vi "FreqSel.vi"(5 "FreqSelRing":u16(ring)=1 items=["0.8 ms", "1.0 ms", "1.6 ms", "3.2 ms", "6.4 ms"]) -> (0 "set sample time [s]":sgl, 1 "actual T_DAQ [ms]":dbl, 2 "f_DAQ [kHz]":dbl, 3 "ModeHex":u16, 4 "FreqHex":u16)   [LabVIEW 2014]
panel:
  out "Hex2Decimal":dbl
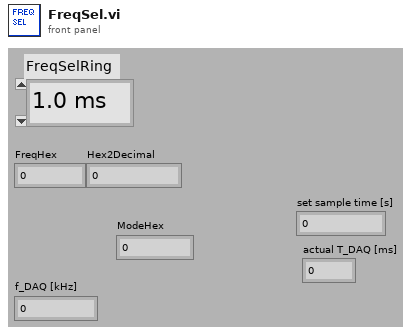
[diagram p1: front panel]
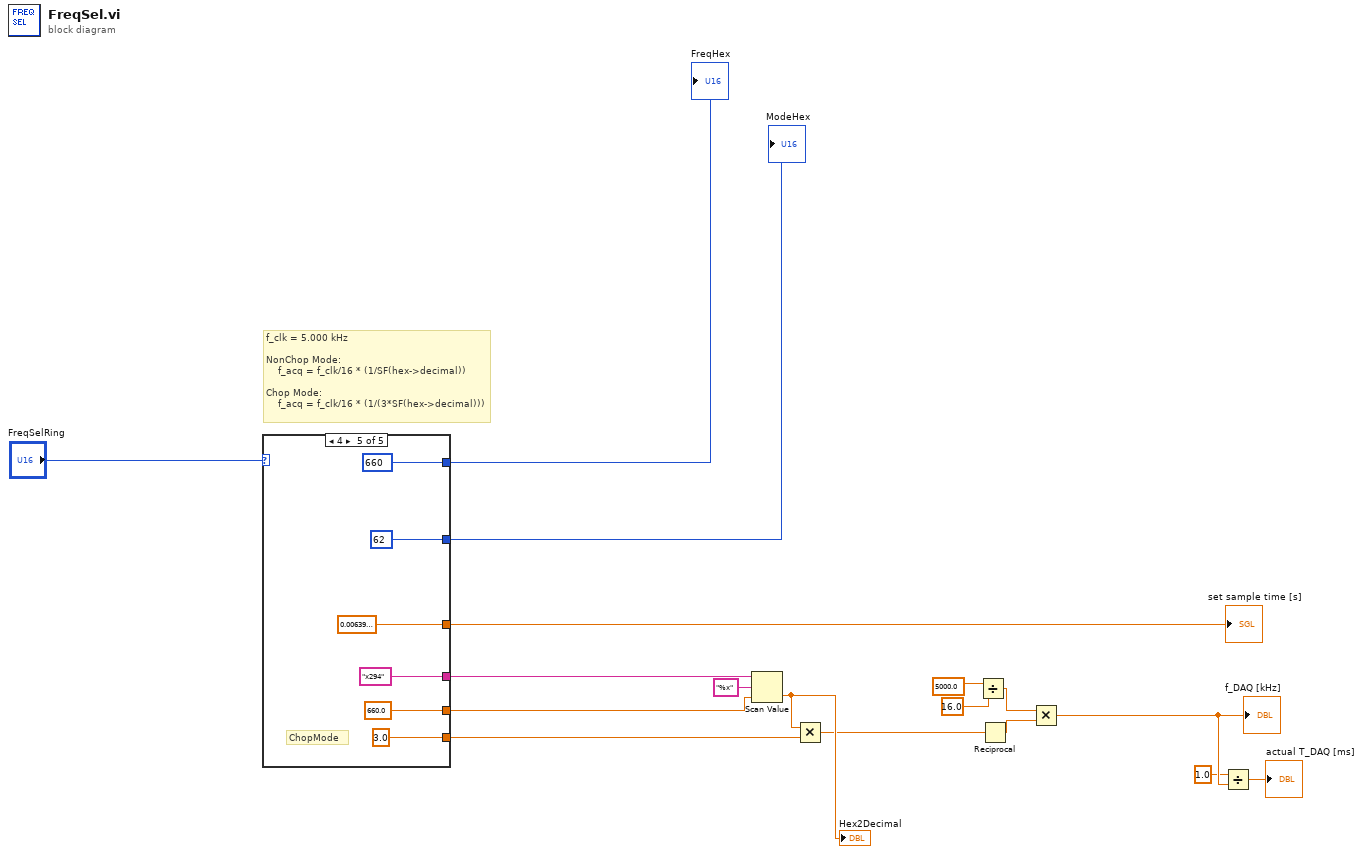
[diagram p0: block diagram]
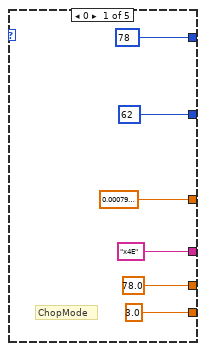
[diagram p2: hidden frame]
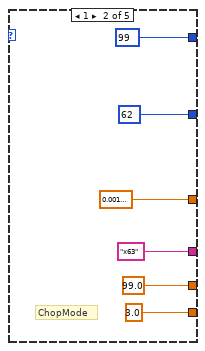
[diagram p3: hidden frame]
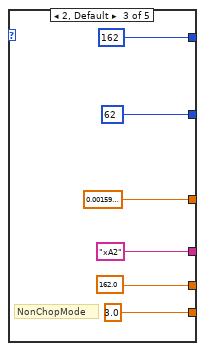
[diagram p4: hidden frame]
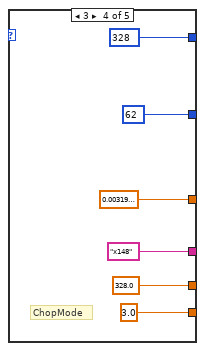
[diagram p5: hidden frame]
diagram:
  # "f_clk = 5.000 kHz\n\nNonChop Mode:\n    f_acq = f_clk/16 * (1/SF(hex->decimal))\n\nChop Mode:\n    f_acq = f_clk/16 * (1/(3*SF(hex->decimal)))"
  n1 = case shown="4" "FreqSelRing" {
    tunnel: [u16 78 ("frequenz") u16 99 ("frequenz") u8 162 ("frequenz") u16 328 ("frequenz") u16 660 ("frequenz")] -> w17
    tunnel: [u16 62 ("t") u16 62 ("t") u16 62 ("t") u16 62 ("t") u16 62 ("t")] -> w16
    tunnel: [sgl 0.0008 sgl 0.001 sgl 0.0016 sgl 0.0032 sgl 0.0064] -> w14
    tunnel: ["x4E" ("string") "x63" ("string") "xA2" ("string") "x148" ("string") "x294" ("string")] -> w3
    tunnel: [78.0 ("default (0 dbl)") 99.0 ("default (0 dbl)") 162.0 ("default (0 dbl)") 328.0 ("default (0 dbl)") 660.0 ("default (0 dbl)")] -> w2
    tunnel: [3.0 ("default (0 dbl)") 3.0 ("default (0 dbl)") 3.0 ("default (0 dbl)") 3.0 ("default (0 dbl)") 3.0 ("default (0 dbl)")] -> w1
    frame 0 {
      # "ChopMode"
    }
    frame 1 {
      # "ChopMode"
    }
    frame 2, Default {
      # "NonChopMode"
    }
    frame 3 {
      # "ChopMode"
    }
    frame 4 {
      # "ChopMode"
    }
  }
  "ModeHex" <- w16
  "FreqHex" <- w17
  "set sample time [s]" <- w14
  n2 = Scan Value(string=w3, format string="%x", default (0 dbl)=w2) -> (value=w13:dbl)  [unwired: 1 out]
  "Hex2Decimal" <- w13
  n3 = Multiply(x=w13, y=w1) -> (x*y=w7:dbl)
  n4 = Divide(x=5000.0 ("default (0 dbl)"), y=16.0 ("default (0 dbl)")) -> (x/y=w9:dbl)
  n5 = Reciprocal(x=w7) -> (1/x=w8:dbl)
  n6 = Multiply(x=w9, y=w8) -> (x*y=w12:dbl)
  "f_DAQ [kHz]" <- w12
  n7 = Divide(x=1.0, y=w12) -> (x/y=→"actual T_DAQ [ms]":dbl)
